vi "UIErrorHandler.vi"(8 "error in (no error)":errorcluster caption="错误输入（无错误）", 10 "error in":errorcluster caption="错误输入（无错误）", 11 "ErrorHanlder 输入":refnum<class "ErrorHanlder.lvclass">) -> (0 "error out":errorcluster caption="错误输出", 3 "ErrorHanlder 输出":refnum<class "ErrorHanlder.lvclass">)   [LabVIEW 2018, in "ErrorHanlder.lvlib" / "ErrorHanlder.lvclass"]
uses:
  ErrorHanlder.lvclass
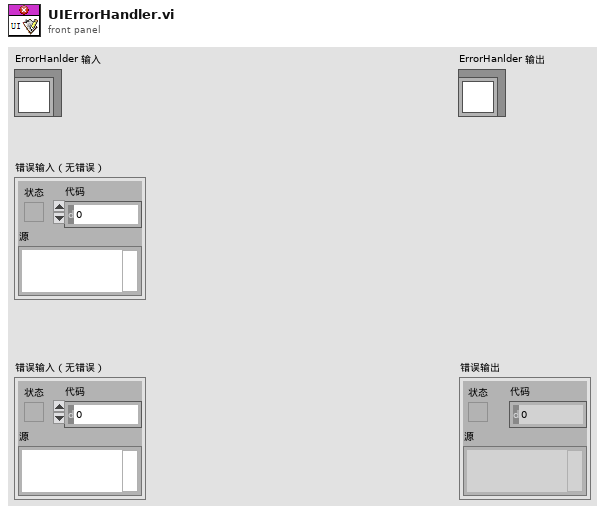
[diagram p1: front panel]
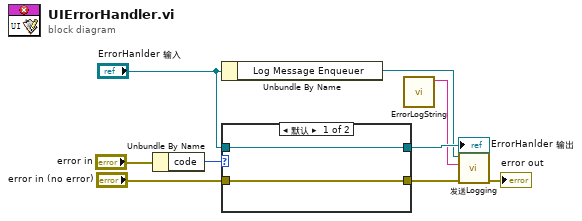
[diagram p0: block diagram]
diagram:
  n1 = Unbundle By Name("error in") -> ("code"=w8:i32)
  n2 = Unbundle By Name("ErrorHanlder 输入") -> ("Log Message Enqueuer"=w2:refnum<class "Message Enqueuer.lvclass">)
  n3 = case shown="默认" w8 {
    tunnel: "error in (no error)" -> [w10 w13]
    tunnel: [w10 w13] -> w1
    tunnel: "ErrorHanlder 输入" -> [w11 w12]
    tunnel: [w11 w12] -> w5
    frame Default {
    }
    frame 0 {
    }
  }
  "ErrorHanlder 输出" <- w5
  n4 = call "ErrorLogString.vi"() -> ("LogString"=w4:string)  [unwired: 10 in, 1 out]
  n5 = call "发送Logging.vi"("error in (no error)"=w1, "Log"=w4, "Message Enqueuer"=w2) -> ("error out"=→"error out":errorcluster)  [unwired: 7 in, 1 out]
